vi "ep_Flicker Block3a.vi"(0 "squared voltage":dbl[](array[numeric]), 1 "init":bool, 5 "nominal frequency":enum16{"50 Hz", "60 Hz"}(ring), 7 "nominal sampling rate [Hz]":dbl=11520.0 format="%0.0f", 9 "input sampling rate":dbl=9600.0) -> (4 "filtered voltage":dbl[](array[numeric]), 10 "output sampling rate":dbl=2400.0)   [LabVIEW 2013, in "NI_EP_Power Quality.lvlib"]
doc: "This VI represent the first filter (of block 3 according IEC 61000-4-15), which eliminates the d.c. and double mains frequency ripple components of the demodulator output."
uses:
  <vilib>/addons/Electrical Power/PQ/NI_EP_Power Quality.lvlib
  <vilib>/Analysis/3filter.llb/Filter Passband Type.ctl
  <vilib>/Analysis/NI_AALBase.lvlib
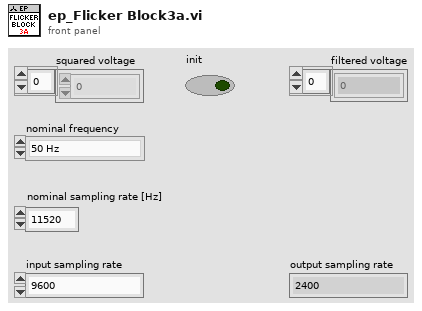
[diagram p1: front panel]
types:
  T1 = typedef "NI_AALBase.lvlib/Filter Passband Type.ctl" = enum32{"Lowpass", "Highpass", "Bandpass", "Bandstop"}
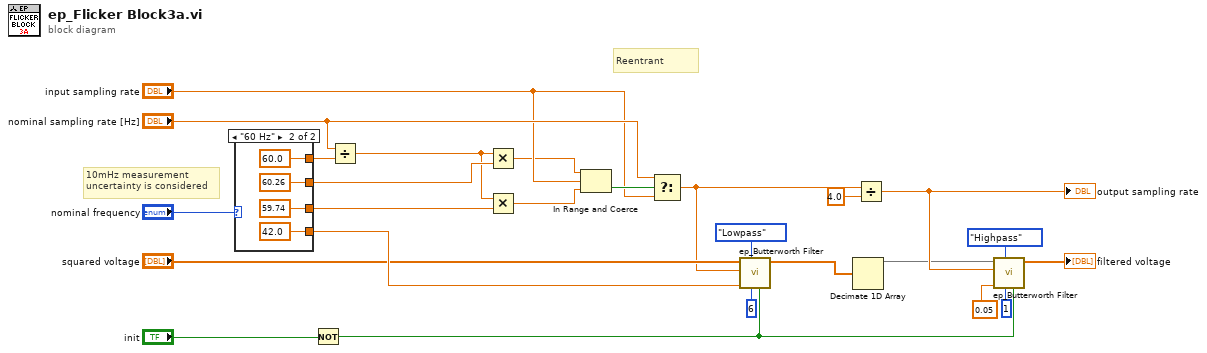
[diagram p0: block diagram]
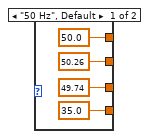
[diagram p2: hidden frame]
diagram:
  # "10mHz measurement\nuncertainty is considered"
  # "Reentrant"
  n1 = case shown="\"60 Hz\"" "nominal frequency" {
    tunnel: [35.0 ("low cutoff freq: fl") 42.0 ("low cutoff freq: fl")] -> w20
    tunnel: [50.0 ("low cutoff freq: fl") 60.0 ("low cutoff freq: fl")] -> w10
    tunnel: [50.26 ("low cutoff freq: fl") 60.26 ("low cutoff freq: fl")] -> w8
    tunnel: [49.74 ("low cutoff freq: fl") 59.74 ("low cutoff freq: fl")] -> w7
    frame "50 Hz", Default {
    }
    frame "60 Hz" {
    }
  }
  n2 = Not(x="init") -> (.not. x?=w14:bool)
  n3 = Divide(x="nominal sampling rate [Hz]", y=w10) -> (x/y=w6:dbl)
  n4 = Multiply(x=w6, y=w8) -> (x*y=w2:dbl)
  n5 = Multiply(x=w6, y=w7) -> (x*y=w1:dbl)
  n6 = In Range and Coerce(upper limit=w2, x="input sampling rate", lower limit=w1) -> (In Range?=w9:bool)  [unwired: 1 out]
  n7 = Select(t="nominal sampling rate [Hz]", s=w9, f="input sampling rate") -> (s? t:f=w4:dbl)
  n8 = call <vilib>:"ep_Butterworth Filter.vi"("init/cont (init:F)"=w14, "order"=6, "filter type"=Filter_Passband_Type."Lowpass", "low cutoff freq: fl"=w20, "sampling freq: fs"=w4, "X"="squared voltage") -> ("Filtered X"=w22:dbl[])  [unwired: 4 in, 1 out]
  n9 = Decimate 1D Array(w22) -> (w23:dbl[])  [unwired: 3 out]
  n10 = Divide(x=w4, y=4.0) -> (x/y=w25:dbl)
  "output sampling rate" <- w25
  n11 = call <vilib>:"ep_Butterworth Filter.vi"("init/cont (init:F)"=w14, "order"=1, "filter type"=Filter_Passband_Type."Highpass", "low cutoff freq: fl"=0.05, "sampling freq: fs"=w25, "X"=w23) -> ("Filtered X"=→"filtered voltage":dbl[])  [unwired: 4 in, 1 out]
